vi "KM_MQM Data Transfer.vi"() -> ()   [LabVIEW 2015]
uses:
  ZI_Frontpanel.ctl
  PPMS_Status.ctl
  Rotator_Status.ctl
  HF_FrontPanel.ctl
panel:
  in  "Tab Control":T1(tab)
  out "ZI HFLI":T2 {"Lockin 1 Demod 0"."R(V)" format="%#_6p"}
  in  "ZI MFLI":T3 {"Lockin 1 Demod 3"."R(V)" format="%#_6p"; "Lockin 1 Demod 2"."R(V)" format="%#_6p"; "Lockin 4 Demod 1"."R(V)" format="%#_6p"; "Lockin 3 Demod 1"."R(V)" format="%#_6p"; "Lockin 2 Demod 1"."R(V)" format="%#_6p"; "Lockin 1 Demod 1"."R(V)" format="%#_6p"; "Lockin 4 Demod 0"."R(V)" format="%#_6p"; "Lockin 3 Demod 0"."R(V)" format="%#_6p"; "Lockin 2 Demod 0"."R(V)" format="%#_6p"; "Lockin 1 Demod 0"."R(V)" format="%#_6p"}
  in  "Keithley":cluster{"Value":dbl, "Keithley on":bool}
  in  "Temperature Control":T4
  in  "System Status":T5
  in  "Rotator":T6
  in  "Magnet parameters":T7={"Max Ramp Rate (T/min)"=0.2, "Max Field (T)"=16.0, "He full"=76.7, "He warning"=50.0, "He low alert"=35.0}
  in  "File Handling":T8 {"Sweep variable" items=["Field", "Temperature", "Angle"]}
  in  "System parameters":cluster{"ZI IP List":string[]}={"ZI IP List"=["192.168.178.11:8004", "192.168.178.12:8004", "192.168.178.13:8004", "192.168.178.14:8004"]}
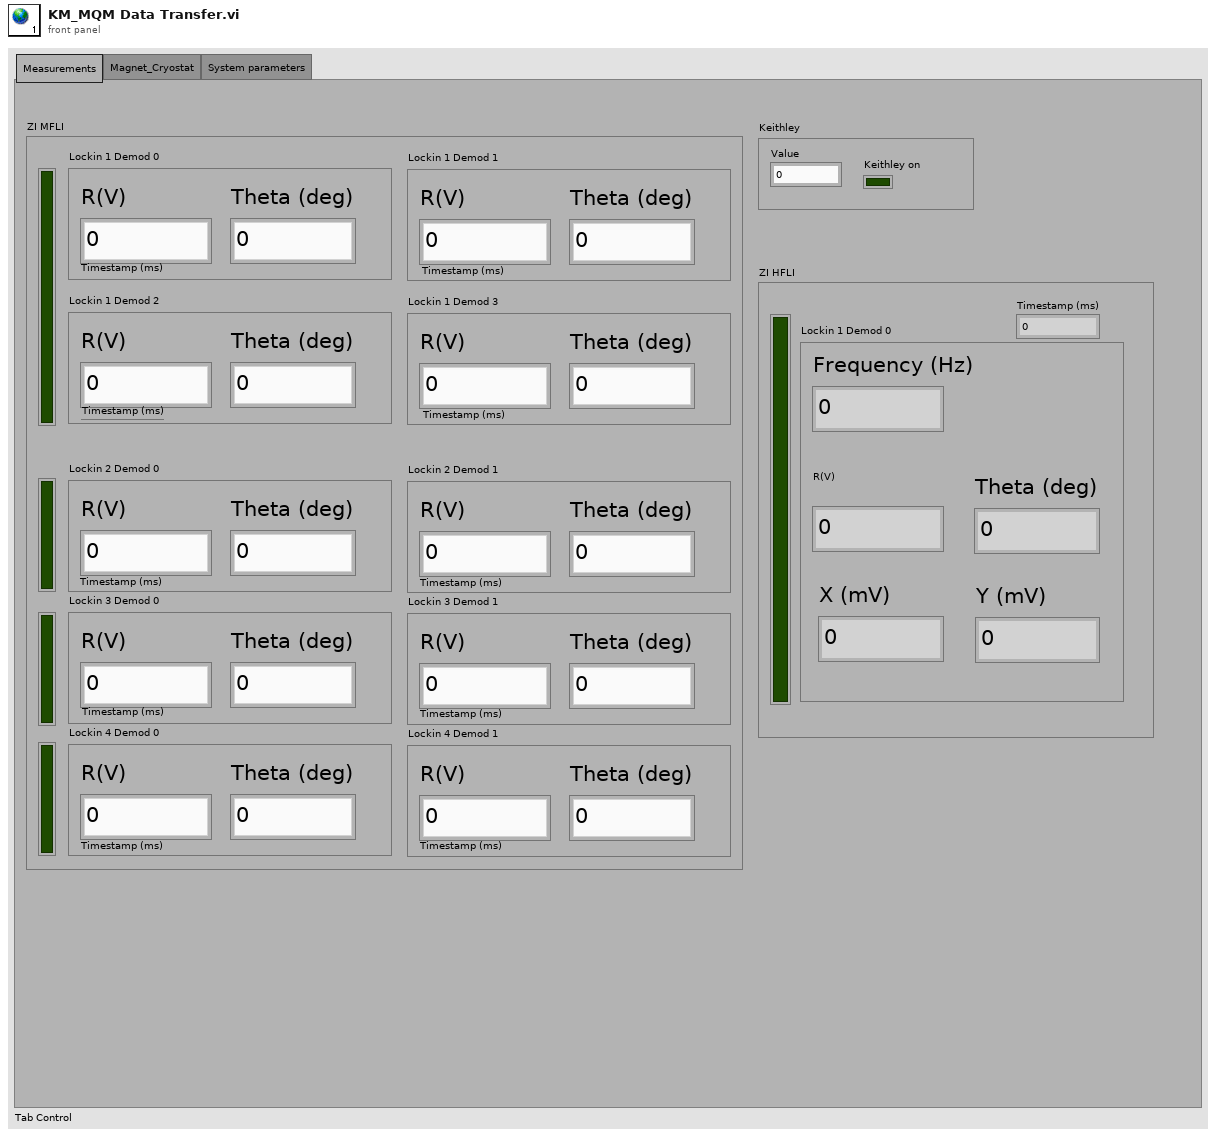
[diagram p1: front panel]
types:
  T1 = enum32{"Measurements", "Magnet_Cryostat", "System parameters"}
  T2 = typedef "HF_FrontPanel.ctl" = cluster{"Lockin 1 Demod 0":cluster{"R(V)":dbl, "Theta (deg)":dbl, "Frequency (Hz)":dbl, "X (mV)":dbl, "Y (mV)":dbl}, "LI1 active":bool, "Timestamp (ms)":u32}
  T3 = typedef "ZI_Frontpanel.ctl" = cluster{"Lockin 1 Demod 0":cluster{"R(V)":dbl, "Theta (deg)":dbl, "Timestamp (ms)":u32}, "Lockin 2 Demod 0":cluster{"R(V)":dbl, "Theta (deg)":dbl, "Timestamp (ms)":u32}, "Lockin 3 Demod 0":cluster{"R(V)":dbl, "Theta (deg)":dbl, "Timestamp (ms)":u32}, "Lockin 4 Demod 0":cluster{"R(V)":dbl, "Theta (deg)":dbl, "Timestamp (ms)":u32}, "Lockin 1 Demod 1":cluster{"R(V)":dbl, "Theta (deg)":dbl, "Timestamp (ms)":u32}, "Lockin 2 Demod 1":cluster{"R(V)":dbl, "Theta (deg)":dbl, "Timestamp (ms)":u32}, "Lockin 3 Demod 1":cluster{"R(V)":dbl, "Theta (deg)":dbl, "Timestamp (ms)":u32}, "Lockin 4 Demod 1":cluster{"R(V)":dbl, "Theta (deg)":dbl, "Timestamp (ms)":u32}, "Lockin 1 Demod 2":cluster{"R(V)":dbl, "Theta (deg)":dbl, "Timestamp (ms)":u32}, "Lockin 1 Demod 3":cluster{"R(V)":dbl, "Theta (deg)":dbl, "Timestamp (ms)":u32}, "LI1 active":bool, "LI2 active":bool, "LI3 active":bool, "LI4 active":bool}
  T4 = cluster{"VTI Setpoint (K)":dbl, "Sample Setpoint (K)":dbl, "Sample Rate (K/min)":dbl, "VTI Ramp Rate (K/min)":dbl, "Temp Control":bool, "Write Setpoints":bool}
  T5 = typedef "PPMS_Status.ctl" = cluster{"Field":cluster{"Field (T)":dbl, "Field stable":bool, "Timestamp (ms)":u32}, "Temperature":cluster{"Temperature (K)":dbl, "Temperature stable":bool, "Timestamp (ms)":u32}}
  T6 = typedef "Rotator_Status.ctl" = cluster{"Angle (deg)":dbl, "Stopped":bool, "Timestamp (ms)":u32}
  T7 = cluster{"Max Ramp Rate (T/min)":dbl, "Max Field (T)":dbl, "He full":dbl, "He warning":dbl, "He low alert":dbl}
  T8 = cluster{"Request new file":bool, "Sweep variable":u16, "Pause DAQ":bool}
diagram:
